vi "MotionMagicDrive.vi"(1 "Enable Vision Y":bool, 4 "X offset":dbl format="%#_13g", 5 "High gear?":bool, 6 "Y offset":dbl format="%#_13g", 7 "Enable Vision X":bool, 8 "error in (no error)":errorcluster, 9 "Y Axis":dbl, 10 "X Axis":dbl, 11 "Pod Drive in":refnum<class "Pod Drive.lvclass">) -> (0 "error out":errorcluster, 3 "Pod Drive out":refnum<class "Pod Drive.lvclass">)   [LabVIEW 2018, in "Drive.lvlib" / "Pod Drive.lvclass"]
doc: "This VI alows you to swich between motion magic GoTo and Closed Loop"
uses:
  Pod Drive.lvclass
  Mode.ctl
  Drive.lvclass
panel:
  in  "Xmultiplyer":dbl=40.0 format="%#_13g"
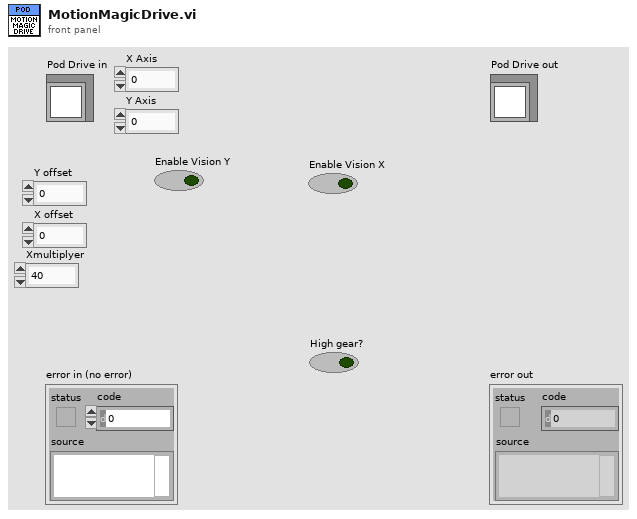
[diagram p1: front panel]
types:
  T1 = typedef "Drive.lvlib/Pod Drive.lvclass/Mode.ctl" = enum16{"ClosedLoop", "MotionMagic"}
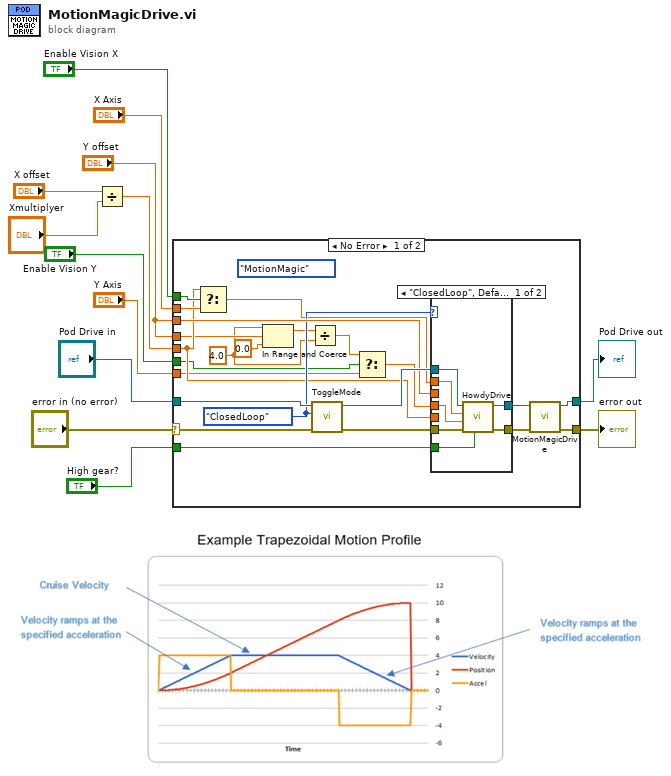
[diagram p0: block diagram]
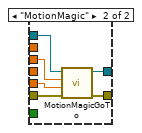
[diagram p2: hidden frame]
diagram:
  n1 = Divide(x="X offset", y="Xmultiplyer") -> (x/y=w4:dbl)
  n2 = case shown="No Error" "error in (no error)" {
    selector: "error in (no error)" -> [w32 w50]
    tunnel: [w36 w50] -> w13
    tunnel: [w35 w51] -> w12
    tunnel: "Pod Drive in" -> [w31 w51]
    tunnel: "Enable Vision X" -> [w24 _]
    tunnel: "Y offset" -> [w29 _]
    tunnel: "X Axis" -> [w28 _]
    tunnel: w4 -> [w23 _]
    tunnel: "Y Axis" -> [w20 _]
    tunnel: "High gear?" -> [w27 _]
    tunnel: "Enable Vision Y" -> [w19 _]
    tunnel: "Y offset" -> [w17 _]
    frame No Error {
      w15 = 4.0 ("upper limit")
      w25 = Mode."ClosedLoop" ("ClosedLoopOrMotionMagic")
      (unwired) Mode."MotionMagic" ("ClosedLoopOrMotionMagic")
      n3 = Select(t=w23, s=w24, f=w28) -> (s? t:f=w22:dbl)
      n4 = In Range and Coerce(upper limit=w15, x=w17, lower limit=0.0) -> (coerced(x)=w16:dbl)  [unwired: 1 out]
      n5 = Divide(x=w16, y=w15) -> (x/y=w14:dbl)
      n6 = call-dynamic "ToggleMode.vi"("error in (no error)"=w32, "Mode"=w25, "Pod Drive in"=w31) -> ("error out"=w26:errorcluster, "Pod Drive out"=w30:refnum<class "Pod Drive.lvclass">)  [unwired: 7 in]
      n7 = Select(t=w14, s=w19, f=w20) -> (s? t:f=w21:dbl)
      n8 = case shown="\"ClosedLoop\", Default" w25 {
        tunnel: w30 -> [w43 w49]
        tunnel: [w42 w48] -> w34
        tunnel: w26 -> [w41 w47]
        tunnel: [w40 w46] -> w33
        tunnel: w29 -> [_ w44]
        tunnel: w23 -> [_ w45]
        tunnel: w21 -> [w38 _]
        tunnel: w22 -> [w39 _]
        tunnel: w27 -> [w37 _]
        frame "ClosedLoop", Default {
          n9 = call-dynamic "HowdyDrive.vi"("HighGear?"=w37, "error in (no error)"=w41, "Y"=w38, "X"=w39, "Pod Drive in"=w43) -> ("error out"=w40:errorcluster, "Pod Drive out"=w42:refnum<class "Pod Drive.lvclass">)  [unwired: 5 in]
        }
        frame "MotionMagic" {
          n10 = call "MotionMagicGoTo.vi"("error in (no error)"=w47, "Offset(deg)"=w45, "Distance(in)"=w44, "Pod Drive in"=w49) -> ("error out"=w46:errorcluster, "Pod Drive out"=w48:refnum<class "Pod Drive.lvclass">)  [unwired: 5 in, 1 out]
        }
      }
      n11 = call-parent "MotionMagicDrive.vi"("error in (no error)"=w33, "Drive in"=w34) -> ("error out"=w36:errorcluster, "Drive out"=w35:refnum<class "Pod Drive.lvclass">)  [unwired: 8 in]
    }
    frame Error {
    }
  }
  "error out" <- w13
  "Pod Drive out" <- w12
